vi "Interpolate Main.vi"(4 "Length":i32, 5 "Data Channels":i32, 7 "NaN":bool, 8 "Sample Rate":i32, 9 "Data":dbl[][](array[numeric]) format="%.2f", 10 "Time":sgl[](array[numeric]) format="%.2f") -> (2 "Interp Data":dbl[][](array[numeric]) format="%.2f")   [LabVIEW 2013]
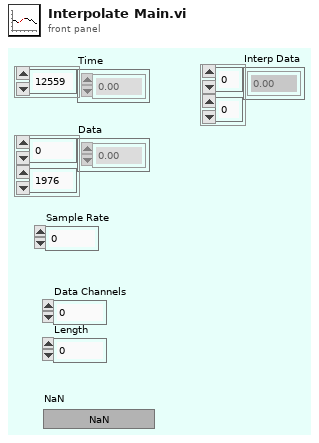
[diagram p1: front panel]
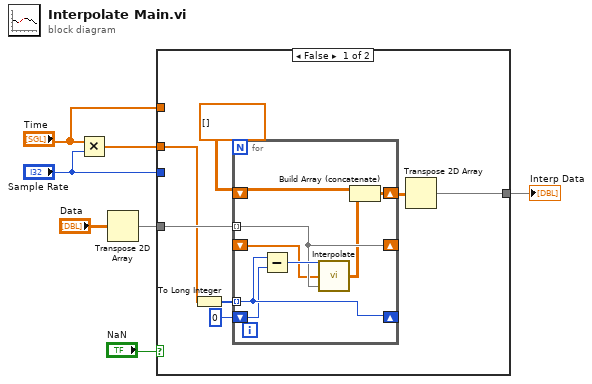
[diagram p0: block diagram]
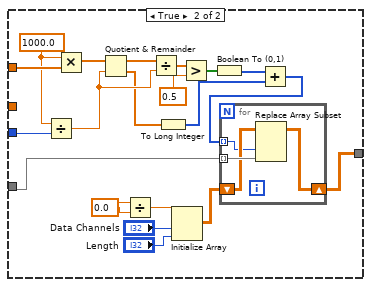
[diagram p2: hidden frame]
diagram:
  n1 = Multiply(x="Time", y="Sample Rate") -> (x*y=w3:sgl[])
  n2 = Transpose 2D Array(2D array="Data") -> (transposed array=w7:dbl[][])
  n3 = case shown="False" "NaN" {
    tunnel: [w14 w36] -> w4
    tunnel: w7 -> [w11 w39]
    tunnel: w3 -> [w8 _]
    tunnel: "Time" -> [_ w35]
    tunnel: "Sample Rate" -> [_ w34]
    frame False {
      n4 = To Long Integer(number=w8) -> (32bit integer=w9:i32[])
      n5 = for {
        tunnel: w9 -> [w22] mode=indexing
        shift-right: [w22] -> _
        shift-left: 0 -> [w21]
        shift-right: [w19] -> _
        shift-left: _ -> [w18]
        tunnel: w11 -> [w19] mode=indexing
        shift-right: [w17] -> w13
        shift-left: dbl[][] [] -> [w15]
        n6 = Subtract(x=w22, y=w21) -> (x-y=w20:i32)
        n7 = call "Interpolate.vi"("Last Scan"=w19, "First Scan"=w18, "Length"=w20) -> ("Ramp Pattern"=w16:dbl[][])
        n8 = Build Array (concatenate)(w15, w16) -> (w17:dbl[][])
      }
      n9 = Transpose 2D Array(2D array=w13) -> (transposed array=w14:dbl[][])
    }
    frame True {
      w33 = 1000.0
      w41 = 0.0
      n10 = Divide(x=w33, y=w34) -> (x/y=w30:dbl)
      n11 = Multiply(x=w33, y=w35) -> (x*y=w32:dbl[])
      n12 = Quotient & Remainder(x=w32, y=w30) -> (x-y*floor(x/y)=w31:dbl[], floor(x/y)=w25:dbl[])
      n13 = Divide(x=w41, y=w41) -> (x/y=w42:dbl)
      n14 = Divide(x=w31, y=w30) -> (x/y=w29:dbl[])
      n15 = To Long Integer(number=w25) -> (32bit integer=w24:i32[])
      n16 = Initialize Array(w42, "Data Channels", "Length") -> (w40:dbl[][])
      n17 = Greater?(x=w29, y=0.5) -> (0:w27:bool[])
      n18 = Boolean To (0,1)(Boolean=w27) -> (0, 1=w26:i16[])
      n19 = Add(x=w26, y=w24) -> (x+y=w23:i32[])
      n20 = for {
        tunnel: w23 -> [w43] mode=indexing
        tunnel: w39 -> [w46] mode=indexing
        shift-right: [w44] -> w36
        shift-left: w40 -> [w45]
        n21 = Replace Array Subset(array=w45, new element=w46, index (col)=w43) -> (w44:dbl[][])  [unwired: 1 in]
      }
    }
  }
  "Interp Data" <- w4
